vi "Save Stim Params.vi"(5 "Right Params":T1, 6 "Left Params":T2, 7 "Stim Parameter Path":path) -> (3 "Stim Parameter Path":path)   [LabVIEW 2019]
uses:
  <vilib>/Utility/file.llb/Write Delimited Spreadsheet (I64).vi
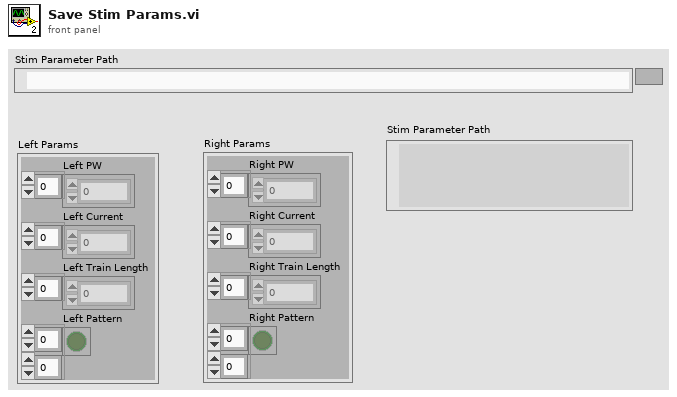
[diagram p1: front panel]
types:
  T1 = cluster{"Right PW":i64[], "Right Current":i64[], "Right Train Length":i64[], "Right Pattern":bool[][]}
  T2 = cluster{"Left PW":i64[], "Left Current":i64[], "Left Train Length":i64[], "Left Pattern":bool[][]}
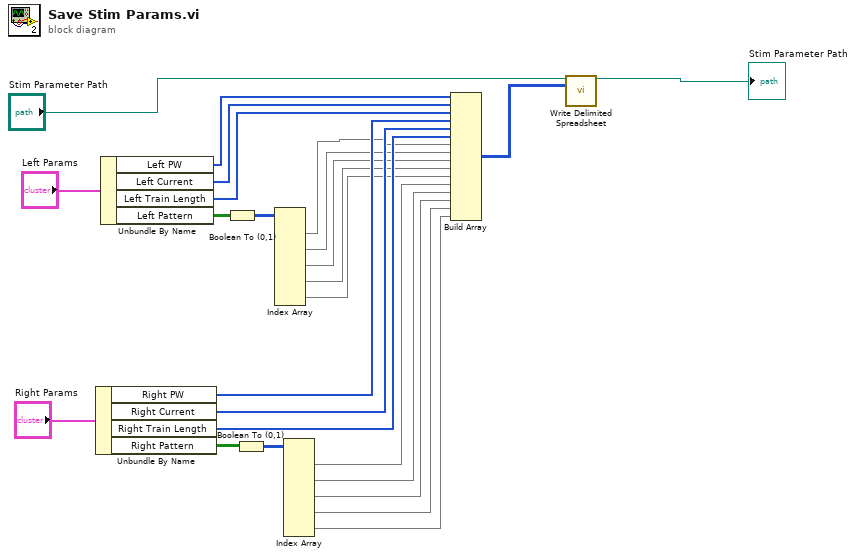
[diagram p0: block diagram]
diagram:
  n1 = Unbundle By Name("Right Params") -> ("Right PW"=w15:i64[], "Right Current"=w14:i64[], "Right Train Length"=w13:i64[], "Right Pattern"=w16:bool[][])
  n2 = Unbundle By Name("Left Params") -> ("Left PW"=w22:i64[], "Left Current"=w21:i64[], "Left Train Length"=w20:i64[], "Left Pattern"=w19:bool[][])
  n3 = Boolean To (0,1)(Boolean=w19) -> (0, 1=w18:i16[][])
  n4 = Boolean To (0,1)(Boolean=w16) -> (0, 1=w17:i16[][])
  n5 = Index Array(array=w18) -> (element #1=w12:i16[], element #2=w11:i16[], element #3=w10:i16[], element #4=w9:i16[], element #5=w8:i16[])  [unwired: 10 in]
  n6 = Index Array(array=w17) -> (element #1=w7:i16[], element #2=w6:i16[], element #3=w5:i16[], element #4=w4:i16[], element #5=w3:i16[])  [unwired: 10 in]
  n7 = Build Array(w22, w21, w20, w15, w14, w13, w12, w11, w10, w9, w8, w7, w6, w5, w4, w3) -> (w2:i64[][])
  n8 = call-poly <vilib>:"Write Delimited Spreadsheet.vi"("file path (dialog if empty)"="Stim Parameter Path", "2D data"=w2) -> ("new file path (Not A Path if cancelled)"=→"Stim Parameter Path":path)  [unwired: 12 in, 1 out]
